vi "Ejemplo1.vi"() -> ()   [LabVIEW 2020]
panel:
  out "Constante":dbl(slide) scale=0.0..100.0
  out "Indicadaor":dbl(slide) scale=0.0..100.0
  in  "Controlador":dbl(slide) scale=0.0..100.0
  # "Panel Frontal"
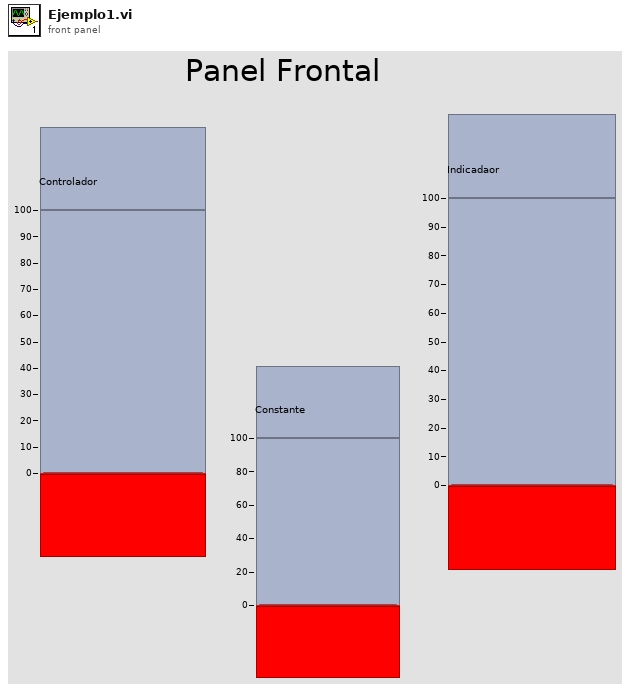
[diagram p1: front panel]
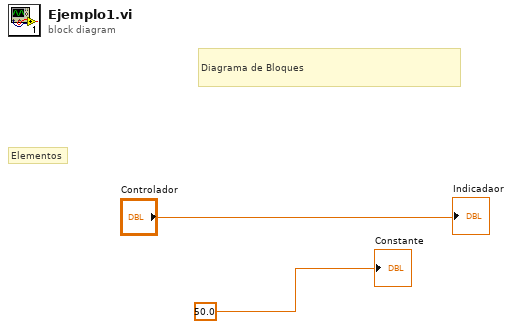
[diagram p0: block diagram]
diagram:
  # "Elementos"
  # "Diagrama de Bloques"
  "Indicadaor" <- "Controlador"
  "Constante" <- 50.0
